vi "Preprocess before printing.vi"(8 "error in (no error)":errorcluster, 11 "Domino Laser module Class in":refnum<class "Domino Laser module Class.lvclass">) -> (0 "error out":errorcluster, 3 "Domino Laser module Class out":refnum<class "Domino Laser module Class.lvclass">)   [LabVIEW 2015, in "Domino LM.lvlib" / "Domino Laser module Class.lvclass"]
uses:
  CTRLS/Domino Laser module Class.lvclass
  CTRLS/Domino Laser module Class.lvclass/Domino Laser module Class.ctl
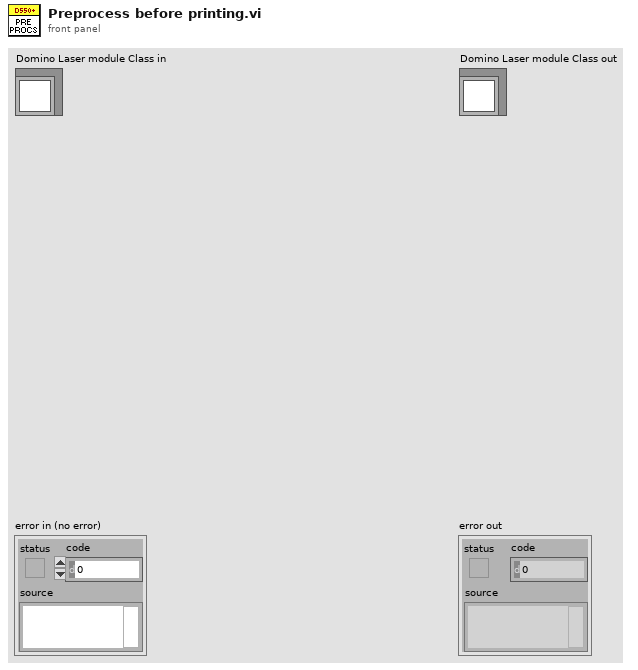
[diagram p1: front panel]
types:
  T1 = cluster{"Layout File":string, "Date Separator":string, "Date Layout":string, "OCR Font":string, "Variable Data":string}
  T2 = typedef "Open Batch Data.ctl" = cluster{"Batch Name":string, "Batch Number":string, "GTIN":string, "Expiry Date":string, "MFG Date":string}
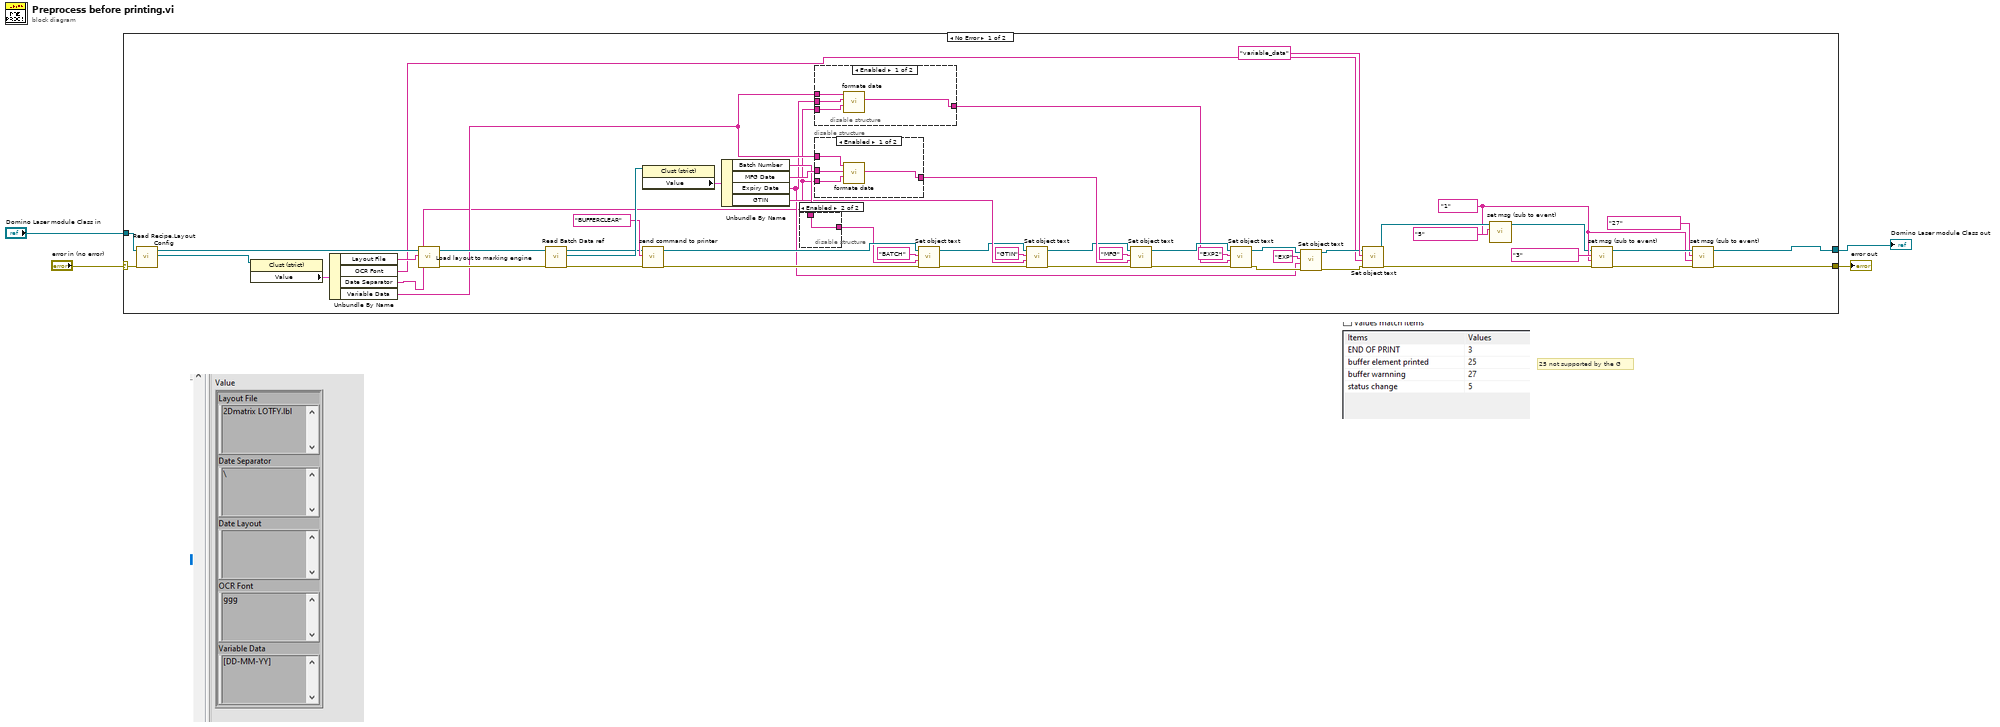
[diagram p0: block diagram]
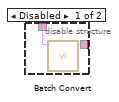
[diagram p2: hidden frame]
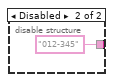
[diagram p3: hidden frame]
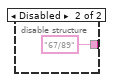
[diagram p4: hidden frame]
diagram:
  # "25 not supported by the G"
  n1 = case shown="No Error" "error in (no error)" {
    selector: "error in (no error)" -> [w46 w71]
    tunnel: [w14 w71] -> w3
    tunnel: [w15 w70] -> w1
    tunnel: "Domino Laser module Class in" -> [w56 w70]
    frame No Error {
      w17 = "1" ("State")
      n2 = call "Read Recipe.Layout Config.vi"("error in (no error)"=w46, "Domino Laser module Class in"=w56) -> ("Recipe.Layout Config"=w55:refnum<vi>, "Domino Laser module Class out"=w47:refnum<class "Domino Laser module Class.lvclass">)  [unwired: 7 in, 1 out]
      n3 = property class="Clust (strict)"(reference=w55) -> ("Value"=w54:T1)  [unwired: 1 in, 2 out]
      n4 = Unbundle By Name(w54) -> ("Layout File"=w53:string, "OCR Font"=w6:string, "Date Separator"=w5:string, "Variable Data"=w13:string)
      n5 = call "Load layout to marking engine.vi"("layout to load"=w53, "Domino Laser module Class in"=w47) -> ("error out"=w51:errorcluster, "Domino Laser module Class out"=w50:refnum<class "Domino Laser module Class.lvclass">)  [unwired: 8 in]
      n6 = call "Read Batch Data ref .vi"("error in (no error)"=w51, "Domino Laser module Class in"=w50) -> ("error out"=w36:errorcluster, "Batch Data"=w49:refnum<vi>, "Domino Laser module Class out"=w41:refnum<class "Domino Laser module Class.lvclass">)  [unwired: 7 in]
      n7 = property class="Clust (strict)"(reference=w49) -> ("Value"=w48:T2)  [unwired: 1 in, 2 out]
      n8 = call "send command to printer.vi"("error in (no error)"=w36, "command to be sent"="BUFFERCLEAR", "Domino Laser module Class in"=w41) -> ("error out"=w35:errorcluster, "Domino Laser module Class out"=w37:refnum<class "Domino Laser module Class.lvclass">)  [unwired: 5 in, 2 out]
      n9 = Unbundle By Name(w48) -> ("Batch Number"=w32:string, "MFG Date"=w40:string, "Expiry Date"=w7:string, "GTIN"=w28:string)
      n10 = disable-structure shown="Enabled" {
        disable-tunnel: w32 -> [w58 w59]
        disable-tunnel: [w57 w59] -> w31
        frame Disabled {
          n11 = call "Batch Convert.vi"("Batch"=w58) -> ("string"=w57:string)  [unwired: 10 in]
        }
        frame Enabled {
        }
      }
      n12 = disable-structure shown="Enabled" {
        disable-tunnel: w5 -> [w68 _]
        disable-tunnel: w13 -> [w67 _]
        disable-tunnel: w7 -> [w66 _]
        disable-tunnel: [w65 "67/89" ("Text")] -> w38
        frame Enabled {
          n13 = call "formate date.vi"("Sepertaor"=w68, "Input Date"=w66, "Layout"=w67) -> ("Formatted Date"=w65:string)  [unwired: 8 in]
        }
        frame Disabled {
        }
      }
      n14 = disable-structure shown="Enabled" {
        disable-tunnel: w40 -> [w63 _]
        disable-tunnel: [w62 "012-345" ("Text")] -> w39
        disable-tunnel: w5 -> [w61 _]
        disable-tunnel: w13 -> [w60 _]
        frame Enabled {
          n15 = call "formate date.vi"("Sepertaor"=w61, "Input Date"=w63, "Layout"=w60) -> ("Formatted Date"=w62:string)  [unwired: 8 in]
        }
        frame Disabled {
        }
      }
      n16 = call "Set object text.vi"("error in (no error)"=w35, "Text"=w31, "Object name"="BATCH", "Domino Laser module Class in"=w37) -> ("error out"=w25:errorcluster, "Domino Laser module Class out"=w26:refnum<class "Domino Laser module Class.lvclass">)  [unwired: 4 in, 2 out]
      n17 = call "Set object text.vi"("error in (no error)"=w25, "Text"=w28, "Object name"="GTIN", "Domino Laser module Class in"=w26) -> ("error out"=w24:errorcluster, "Domino Laser module Class out"=w23:refnum<class "Domino Laser module Class.lvclass">)  [unwired: 4 in, 2 out]
      n18 = call "Set object text.vi"("error in (no error)"=w24, "Text"=w39, "Object name"="MFG", "Domino Laser module Class in"=w23) -> ("error out"=w43:errorcluster, "Domino Laser module Class out"=w45:refnum<class "Domino Laser module Class.lvclass">)  [unwired: 4 in, 2 out]
      n19 = call "Set object text.vi"("error in (no error)"=w43, "Text"=w38, "Object name"="EXP2", "Domino Laser module Class in"=w45) -> ("error out"=w9:errorcluster, "Domino Laser module Class out"=w8:refnum<class "Domino Laser module Class.lvclass">)  [unwired: 4 in, 2 out]
      n20 = call "Set object text.vi"("error in (no error)"=w9, "Text"=w7, "Object name"="EXP", "Domino Laser module Class in"=w8) -> ("error out"=w10:errorcluster, "Domino Laser module Class out"=w11:refnum<class "Domino Laser module Class.lvclass">)  [unwired: 4 in, 2 out]
      n21 = call "Set object text.vi"("error in (no error)"=w10, "Text"=w6, "Object name"="variable_data", "Domino Laser module Class in"=w11) -> ("error out"=w34:errorcluster, "Domino Laser module Class out"=w30:refnum<class "Domino Laser module Class.lvclass">)  [unwired: 4 in, 2 out]
      n22 = call "set msg (sub to event).vi"("State"=w17, "MSG"="5", "Domino Laser module Class in"=w30) -> ("Domino Laser module Class out"=w16:refnum<class "Domino Laser module Class.lvclass">)  [unwired: 7 in, 1 out]
      n23 = call "set msg (sub to event).vi"("error in (no error)"=w34, "State"=w17, "MSG"="3", "Domino Laser module Class in"=w16) -> ("error out"=w19:errorcluster, "Domino Laser module Class out"=w21:refnum<class "Domino Laser module Class.lvclass">)  [unwired: 6 in]
      n24 = call "set msg (sub to event).vi"("error in (no error)"=w19, "State"=w17, "MSG"="27", "Domino Laser module Class in"=w21) -> ("error out"=w14:errorcluster, "Domino Laser module Class out"=w15:refnum<class "Domino Laser module Class.lvclass">)  [unwired: 6 in]
    }
    frame Error {
    }
  }
  "error out" <- w3
  "Domino Laser module Class out" <- w1
